vi "GetChoreoDt.vi"(9 "index":dbl, 10 "dt array":dbl[](array[numeric])) -> (1 "Choreo Path?":bool, 2 "dt":dbl)   [LabVIEW 2025]
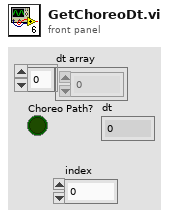
[diagram p1: front panel]
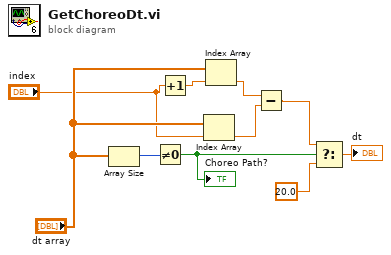
[diagram p0: block diagram]
diagram:
  n1 = Array Size(array="dt array") -> (size(s)=w10:i32)
  n2 = Not Equal To 0?(x=w10) -> (x != 0?=w4:bool)
  "Choreo Path?" <- w4
  n3 = Increment(x="index") -> (x+1=w8:dbl)
  n4 = Index Array(array="dt array", index="index") -> (element=w5:dbl)
  n5 = Index Array(array="dt array", index=w8) -> (element=w6:dbl)
  n6 = Subtract(x=w6, y=w5) -> (x-y=w2:dbl)
  n7 = Select(t=w2, s=w4, f=20.0) -> (s? t:f=→"dt":dbl)
